vi "example-TextControlledInstrum.vi"() -> ()   [LabVIEW 2020]
uses:
  TextControlledInstrumIOQueuePacket.ctl
  TextControlledInstrum/TextControlledInstrumCommandsToArraySingle.vi
panel:
  in  "Serial port":refnum<visa-resource-name>="COM7"
  in  "Cluster":T1
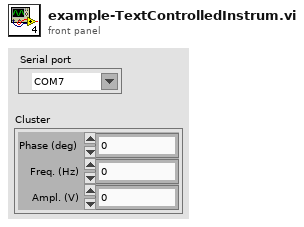
[diagram p1: front panel]
types:
  T1 = cluster{"Phase (deg)":dbl, "Freq. (Hz)":dbl, "Ampl. (V)":dbl}
  T2 = typedef "TextControlledInstrumIOQueuePacket.ctl" = cluster{"Operation":enum16{"read", "write", "reserved2", "reserved3", "reserved4", "reserved5", "reserved6", "reserved7"}, "Data":string, "Queue":refnum<queue>}
  T3 = map{refnum<vi>, cluster{"Index":i32, "Length":i32}}
  T4 = enum16{"read", "write", "reserved2", "reserved3", "reserved4", "reserved5", "reserved6", "reserved7"}
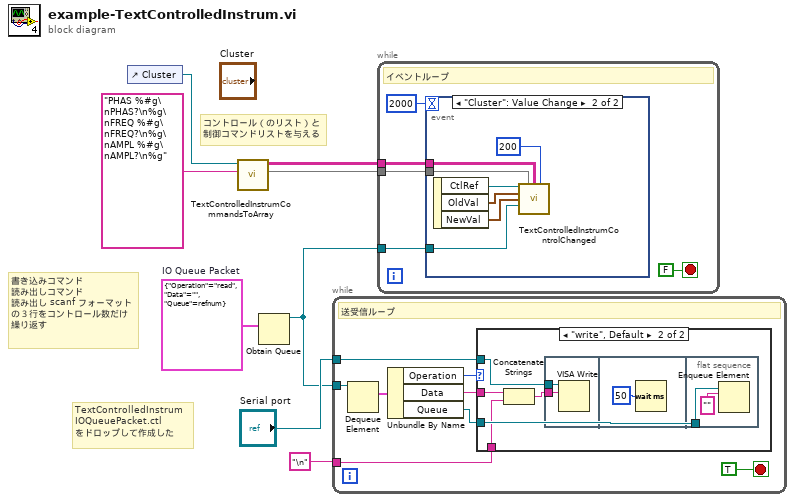
[diagram p0: block diagram]
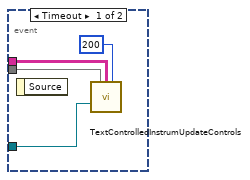
[diagram p2: hidden frame]
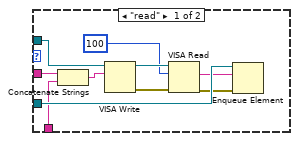
[diagram p3: hidden frame]
diagram:
  w5 = T2 {"Operation"=enum."read", "Data"="", "Queue"=refnum}  # IO Queue Packet
  # "書き込みコマンド\n読み出しコマンド\n読み出し scanf フォーマット\nの３行をコントロール数だけ\n繰り返す"
  # "コントロール（のリスト）と\n制御コマンドリストを与える"
  # "TextControlledInstrum\nIOQueuePacket.ctl\nをドロップして作成した"
  n1 = control-ref of="Cluster"() -> (w7:refnum<vi>)
  n2 = call-poly "TextControlledInstrumCommandsToArray.vi"("SetGetCommands"="PHAS %#g\nPHAS?\n%g\nFREQ %#g\nFREQ?\n%g\nAMPL %#g\nAMPL?\n%g", "Control"=w7) -> ("Control to Index"=w2:T3, "Command Array"=w3:string[][])  [unwired: 8 in]
  n3 = Obtain Queue(element data type=w5) -> (queue out=w4:refnum<queue>)  [unwired: 4 in, 2 out]
  n4 = while {
    tunnel: "Serial port" -> [w14]
    tunnel: w4 -> [w13]
    tunnel: "\n" ("string") -> [w9]
    stop <- TRUE stop-if-true
    # "送受信ループ"
    n5 = Dequeue Element(queue=w13) -> (element=w16:T2)  [unwired: 2 in, 3 out]
    n6 = Unbundle By Name(w16) -> ("Operation"=w11:T4, "Data"=w10:string, "Queue"=w12:refnum<queue>)
    n7 = case shown="\"write\", Default" w11 {
      tunnel: w10 -> [w25 w29]
      tunnel: w12 -> [w22 w31]
      tunnel: w14 -> [w26 w30]
      tunnel: w9 -> [w17 w27]
      frame "read" {
        n8 = Concatenate Strings(w25, w17) -> (w18:string)
        n9 = VISA Write(VISA resource name=w26, write buffer=w18) -> (VISA resource name out=w23:refnum<visa-resource-name>, error out=w24:errorcluster)  [unwired: 1 in, 1 out]
        n10 = VISA Read(VISA resource name=w23, byte count=u32 100, error in (no error)=w24) -> (read buffer=w21:string, error out=w20:errorcluster)  [unwired: 2 out]
        n11 = Enqueue Element(queue=w22, element=w21, error in (no error)=w20) -> ()  [unwired: 1 in, 3 out]
      }
      frame "write", Default {
        n12 = Concatenate Strings(w29, w27) -> (w28:string)
        n13 = flat-sequence {
          tunnel: w30 -> [w33]
          tunnel: w28 -> [w32]
          tunnel: w31 -> [w36]
          frame #0 {
            n14 = VISA Write(VISA resource name=w33, write buffer=w32) -> ()  [unwired: 1 in, 3 out]
          }
          frame #1 {
            n15 = Wait (ms)(milliseconds to wait=u32 50) -> ()  [unwired: 1 out]
          }
          frame #2 {
            n16 = Enqueue Element(queue=w36, element="") -> ()  [unwired: 2 in, 3 out]
          }
        }
      }
    }
  }
  n17 = while {
    tunnel: w4 -> [w39]
    tunnel: w3 -> [w38]
    tunnel: w2 -> [w37]
    stop <- FALSE stop-if-true
    # "イベントループ"
    n18 = event shown="[1] \"Cluster\": Value Change" {
      selector: _ -> [_ _]
      dyn-events: _ -> [_ _]
      timeout: 2000 -> [_ _]
      tunnel: w39 -> [w45 w52]
      tunnel: w38 -> [w44 w47]
      tunnel: w37 -> [w43 w48]
      event Timeout {
        n19 = event-data() -> ()  [unwired: 1 in, 1 out]
        n20 = call "TextControlledInstrumUpdateControls.vi"("Control To Index"=w43, "Command Array"=w44, "timeout in ms (1000ms)"=200, "IO Queue"=w45) -> ()  [unwired: 12 in]
      }
      event "Cluster": Value Change {
        n21 = event-data() -> ("CtlRef"=w49:refnum<vi>, "OldVal"=w50:T1, "NewVal"=w51:T1)  [unwired: 1 in]
        n22 = call "TextControlledInstrumControlChanged.vi"("CtlRef"=w49, "Control to Index"=w48, "Command Array"=w47, "timeout in ms (1000ms)"=200, "OldVal"=w50, "NewVal"=w51, "IO Queue"=w52) -> ()  [unwired: 9 in]
      }
    }
  }
